vi "Pre-Build Action.vi"(6 "Top Level/Always Included VIs":path[](array[path]), 7 "Main Destination Path":path, 9 "Target Name":string, 10 "Build Specification Name":string, 11 "Project Path":path=path "C:/LabVIEW Code/TALOS/talos/TALOS.lvproj") -> (0 "error out":errorcluster)   [LabVIEW 2026]
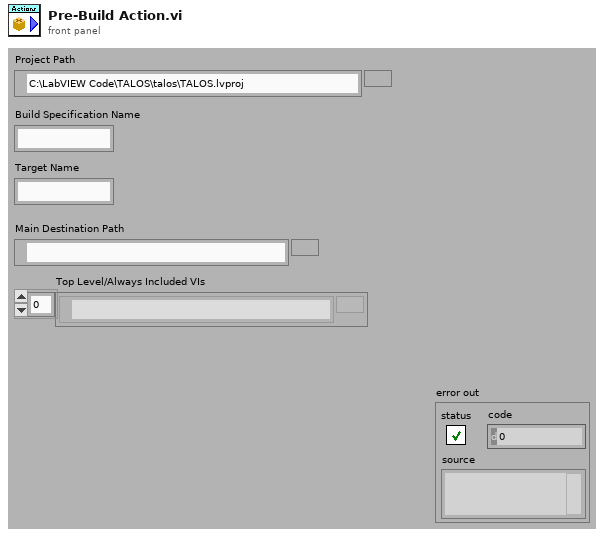
[diagram p1: front panel]
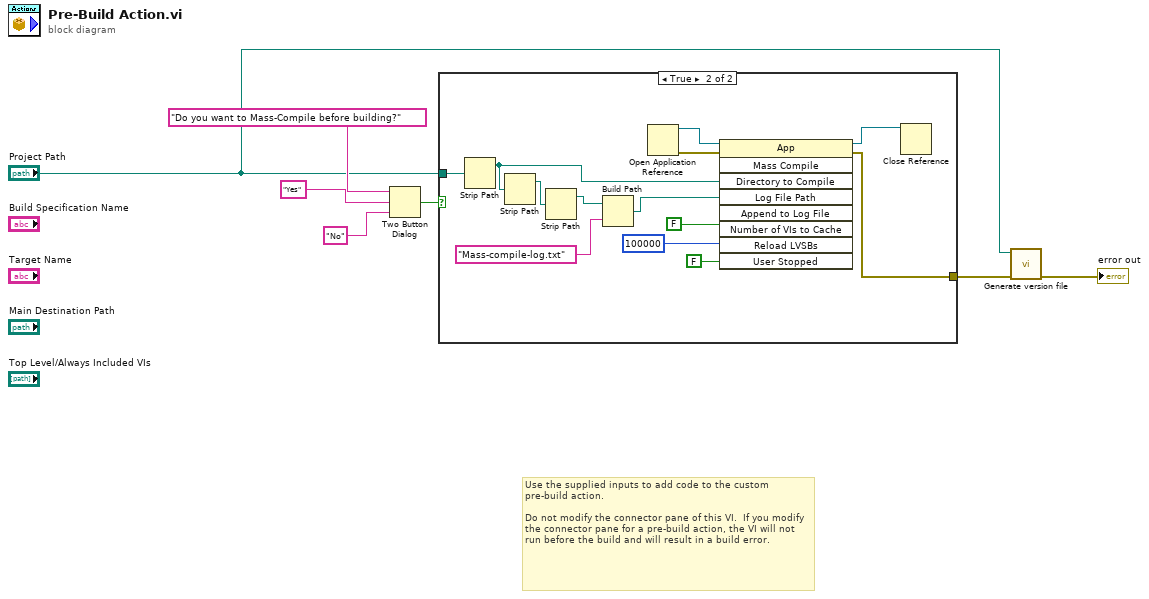
[diagram p0: block diagram]
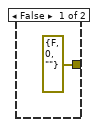
[diagram p2: hidden frame]
diagram:
  # "Use the supplied inputs to add code to the custom pre-build action.\n\nDo not modify the connector pane of this VI.  If you modify the connector pane for a pre-build action, the VI will not run before the build and will result in a build error."
  n1 = Two Button Dialog(message="Do you want to Mass-Compile before building?", 1:"No" ("F button name (\"Cancel\")"), 2:"Yes" ("T button name (\"OK\")")) -> (T button?=w7:bool)
  n2 = case shown="True" w7 {
    tunnel: "Project Path" -> [_ w19]
    tunnel: [errorcluster {"status"=FALSE, "code"=0, "source"=""} ("error out") w13] -> w2
    frame False {
    }
    frame True {
      n3 = Strip Path(path=w19) -> (stripped path=w16:path)  [unwired: 1 out]
      n4 = Strip Path(path=w16) -> (stripped path=w10:path)  [unwired: 1 out]
      n5 = Strip Path(path=w10) -> (stripped path=w9:path)  [unwired: 1 out]
      n6 = Build Path(base path=w9, name or relative path="Mass-compile-log.txt") -> (appended path=w14:path)
      n7 = Open Application Reference() -> (0:w20:errorcluster, 3:w21:refnum<vi>)  [unwired: 4 in]
      n8 = invoke class="App" method="Mass Compile"(reference=w21, error in=w20, "Directory to Compile"=w16, "Log File Path"=w14, "Append to Log File"=FALSE, "Number of VIs to Cache"=u32 100000, "Reload LVSBs"=FALSE) -> (reference out=w12:refnum<vi>, error out=w13:errorcluster)  [unwired: 2 in, 7 out]
      n9 = Close Reference(reference=w12) -> ()  [unwired: 1 in, 1 out]
    }
  }
  n10 = call "Generate version file.vi"("error in (no error)"=w2, "Project Path"="Project Path") -> ("error out"=→"error out":errorcluster)  [unwired: 9 in]
